vi "Initializer.vi"(8 "Error In":errorcluster, 10 "Display Table Ref":refnum<vi>, 11 "Configuration Table Ref":refnum<vi>) -> (0 "Error Out":errorcluster)   [LabVIEW 2014]
uses:
  Controls/FGVisfileopen.ctl
panel:
  in  "Table":i32(listbox)
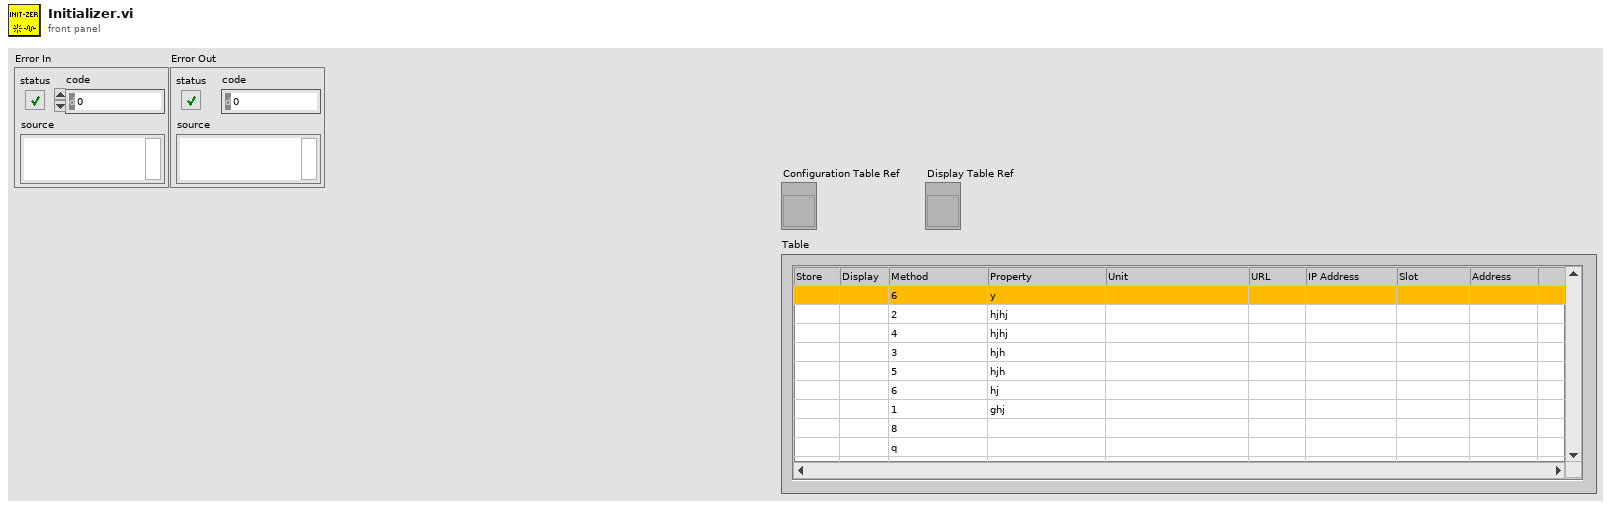
[diagram p1: front panel]
types:
  T1 = typedef "FGVisfileopen.ctl" = enum16{"Read", "Write"}
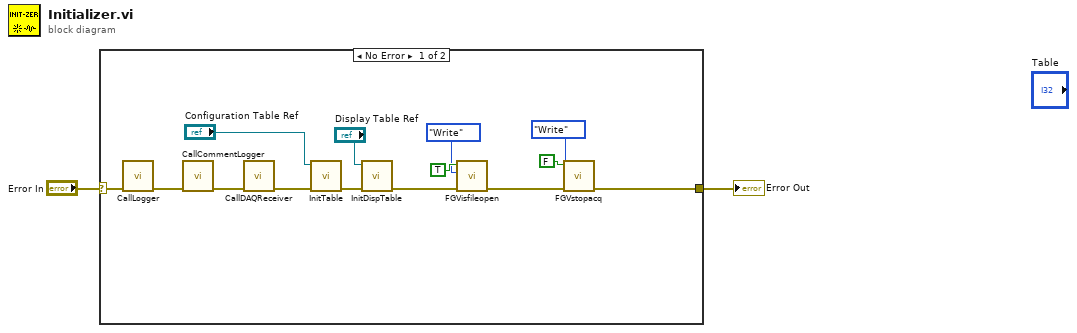
[diagram p0: block diagram]
diagram:
  n1 = case shown="No Error" "Error In" {
    selector: "Error In" -> [w3 w17]
    tunnel: [w4 w17] -> w2
    frame No Error {
      n2 = call "CallLogger.vi"("error in"=w3) -> ("error out"=w14:errorcluster)  [unwired: 10 in]
      n3 = call "CallCommentLogger.vi"("error in"=w14) -> ("error out"=w12:errorcluster)  [unwired: 10 in]
      n4 = call "CallDAQReceiver.vi"("error in"=w12) -> ("error out"=w11:errorcluster)  [unwired: 10 in]
      n5 = call "InitTable.vi"("Error In"=w11, "Table 2"="Configuration Table Ref") -> ("Error Out"=w7:errorcluster)  [unwired: 9 in]
      n6 = call "InitDispTable.vi"("Error In"=w7, "Table Display"="Display Table Ref") -> ("Error Out"=w6:errorcluster)  [unwired: 9 in]
      n7 = call "FGVisfileopen.vi"("error in"=w6, "Read/Write?"=FGVisfileopen."Write" ("Write from FGV or Read from FGV?"), "Input Value"=TRUE) -> ("error out"=w8:errorcluster)  [unwired: 7 in, 1 out]
      n8 = call "FGVstopacq.vi"("error in"=w8, "Write from FGV or Read from FGV?"=FGVisfileopen."Write", "Input Value"=FALSE) -> ("error out"=w4:errorcluster)  [unwired: 7 in, 1 out]
    }
    frame Error {
    }
  }
  "Error Out" <- w2
